vi "SFID Get Nsamples.vi"(3 "N samples":u32=1000, 4 "Data rate (Hz) In":dbl=100.0 format="%#_13g", 5 "COM port":refnum<visa-resource-name>) -> (0 "Error out":errorcluster, 1 "Data rate (Hz) Out":dbl=100.0, 2 "Voltage array out":sgl[](array[numeric]))   [LabVIEW 2022 SP3]
uses:
  Ctls/SFID_Cmd.ctl
panel:
  in  "Stop Button":bool
  out "Data chart":cluster{"Vout (V)":sgl}(graph)
  # "Data rate = 100 Hz"
  # "Vout (V)"
  # "Surrey Sensors 08/2024  v1.0"
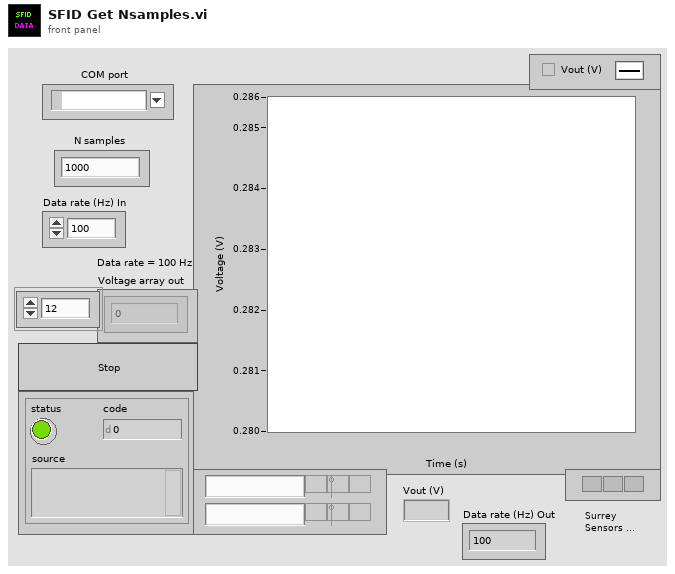
[diagram p1: front panel]
types:
  T1 = typedef "SFID_Cmd.ctl" = string
  T2 = typedef "SFID_Data.ctl" = cluster{"Vout (V)":sgl}
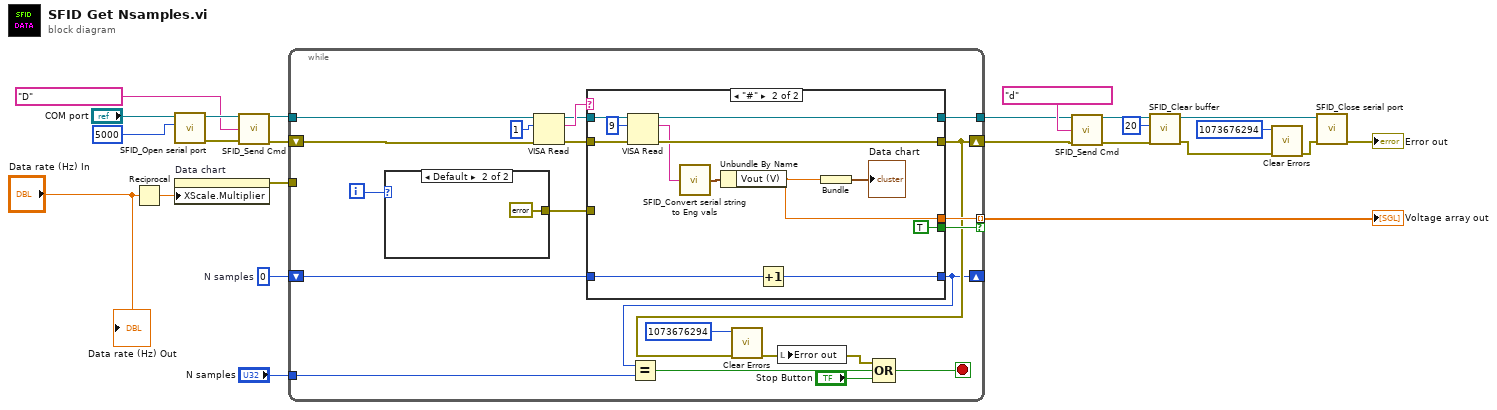
[diagram p0: block diagram]
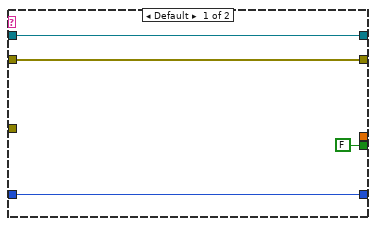
[diagram p2: hidden frame]
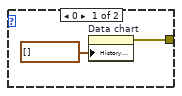
[diagram p3: hidden frame]
diagram:
  w3 = u32 0  # N samples
  n1 = Reciprocal(x="Data rate (Hz) In") -> (1/x=w9:dbl)
  n2 = call "SFID_Open serial port.vi"("timeout (ms)"=u32 5000, "VISA resource name"="COM port") -> ("Error out"=w14:errorcluster, "VISA resource name out"=w16:refnum<visa-resource-name>)  [unwired: 8 in]
  n3 = property on="Data chart" class="WFChart (strict)"("XScale.Multiplier"=w9) -> (error out=w11:errorcluster)  [unwired: 2 in, 1 out]
  n4 = call "SFID_Send Cmd.vi"("Port"=w16, "Cmd"=T1 "D", "Error In"=w14) -> ("Port out"=w13:refnum<visa-resource-name>, "Error Out"=w12:errorcluster)  [unwired: 11 in]
  n5 = while {
    shift-right: [w32] -> w17
    shift-left: w12 -> [w37]
    tunnel: w11 -> [_]
    tunnel: w13 -> [w38]
    tunnel: [w40] -> w18
    shift-right: [w29] -> _
    shift-left: w3 -> [w36]
    tunnel: [w35] -> w2 mode=indexing if=w34
    tunnel: "N samples" -> [w30]
    i -> [w25]
    stop <- w28 stop-if-true
    n6 = case shown="Default" w25 {
      tunnel: [w62 errorcluster {"status"=FALSE, "code"=0, "source"=""} ("error out")] -> w39
      frame 0 {
        n7 = property on="Data chart" class="WFChart (strict)"("History Data"=cluster{"Vout (V)":sgl}[] []) -> (error out=w62:errorcluster)  [unwired: 2 in, 1 out]
      }
      frame Default {
      }
    }
    n8 = VISA Read(VISA resource name=w38, byte count=u32 1, error in (no error)=w37) -> (VISA resource name out=w42:refnum<visa-resource-name>, read buffer=w43:string, error out=w41:errorcluster)  [unwired: 1 out]
    n9 = case shown="\"#\"" w43 {
      tunnel: w42 -> [w47 w60]
      tunnel: w41 -> [w48 w59]
      tunnel: [w47 w57] -> w40
      tunnel: [w48 w56] -> w32
      tunnel: w39 -> [_ _]
      tunnel: w36 -> [w46 w52]
      tunnel: [w46 w51] -> w29
      tunnel: [_ w49] -> w35
      tunnel: [FALSE TRUE] -> w34
      frame Default {
      }
      frame "#" {
        n10 = VISA Read(VISA resource name=w60, byte count=u32 9, error in (no error)=w59) -> (VISA resource name out=w57:refnum<visa-resource-name>, read buffer=w55:string, error out=w56:errorcluster)  [unwired: 1 out]
        n11 = call "SFID_Convert serial string to Eng vals.vi"("Serial buffer string (excluding FrameChar)"=w55) -> ("SFID data"=w54:T2)
        n12 = Unbundle By Name(w54) -> ("Vout (V)"=w49:sgl)
        n13 = Increment(x=w52) -> (x+1=w51:u32)
        n14 = Bundle("Vout (V)"=w49) -> (→"Data chart":cluster{"Vout (V)":sgl})  [unwired: 1 in]
      }
    }
    n15 = Equal?(x=w29, y=w30) -> (x = y?=w27:bool)
    n16 = call <vilib>:"Clear Errors.vi"("error in (no error)"=w32, "specific error code to clear (0: all)"=1073676294) -> ("error out"=w31:errorcluster)  [unwired: 4 in, 1 out]
    n17 = local write "Error out"(w31) -> ()
    n18 = Compound Arithmetic op=OR(w31, w27, "Stop Button") -> (w28:bool)
  }
  "Voltage array out" <- w2
  n19 = call "SFID_Send Cmd.vi"("Port"=w18, "Cmd"=T1 "d", "Error In"=w17) -> ("Port out"=w5:refnum<visa-resource-name>, "Error Out"=w4:errorcluster)  [unwired: 11 in]
  n20 = call "SFID_Clear buffer.vi"("Error in"=w4, "dt for timeout (ms)"=u32 20, "VISA resource name in"=w5) -> ("Error out"=w6:errorcluster, "VISA resource name out"=w7:refnum<visa-resource-name>)  [unwired: 3 in]
  n21 = call <vilib>:"Clear Errors.vi"("error in (no error)"=w6, "specific error code to clear (0: all)"=1073676294) -> ("error out"=w21:errorcluster)  [unwired: 4 in, 1 out]
  n22 = call "SFID_Close serial port.vi"("Error in"=w21, "VISA resource name"=w7) -> ("Error out"=→"Error out":errorcluster)  [unwired: 9 in]
  "Data rate (Hz) Out" <- "Data rate (Hz) In"
